vi "Arduino - Sensor shape data.vi"(8 "Error In":errorcluster, 10 "Sensor Data in":dbl[](array[numeric])) -> (0 "Error Out":errorcluster, 2 "Sensor Data Out":T1)   [LabVIEW 2014]
uses:
  Typedef/sensor_data.ctl
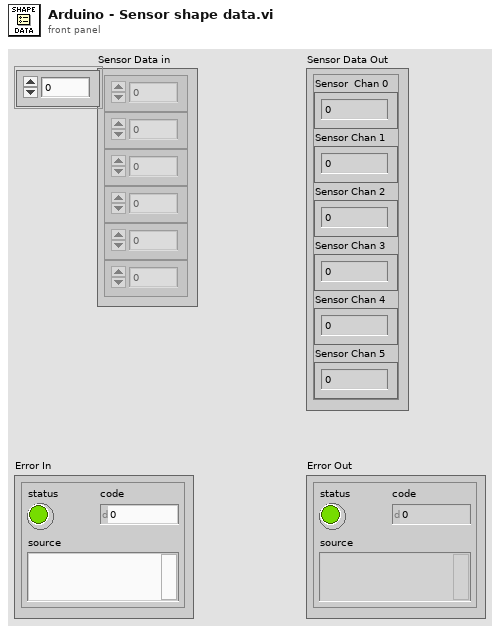
[diagram p1: front panel]
types:
  T1 = typedef "Sensor_data.ctl" = cluster{"Sensor  Chan 0":dbl, "Sensor Chan 1":dbl, "Sensor Chan 2":dbl, "Sensor Chan 3":dbl, "Sensor Chan 4":dbl, "Sensor Chan 5":dbl}
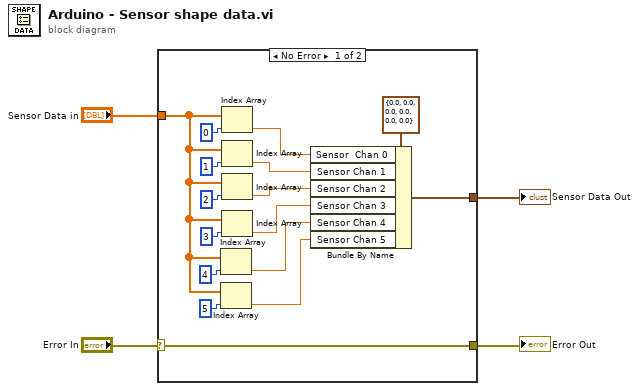
[diagram p0: block diagram]
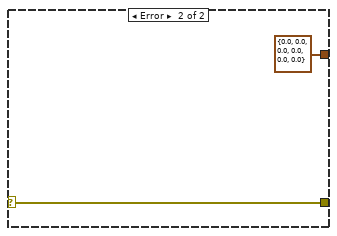
[diagram p2: hidden frame]
diagram:
  n1 = case shown="No Error" "Error In" {
    selector: "Error In" -> [w5 w21]
    tunnel: [w13 T1 {"Sensor  Chan 0"=0.0, "Sensor Chan 1"=0.0, "Sensor Chan 2"=0.0, "Sensor Chan 3"=0.0, "Sensor Chan 4"=0.0, "Sensor Chan 5"=0.0} ("Sensor Data")] -> w4
    tunnel: "Sensor Data in" -> [w12 _]
    tunnel: [w5 w21] -> w1
    frame No Error {
      n2 = Index Array(array=w12, index=4) -> (element=w7:dbl)
      n3 = Index Array(array=w12, index=5) -> (element=w6:dbl)
      n4 = Index Array(array=w12, index=0) -> (element=w11:dbl)
      n5 = Index Array(array=w12, index=1) -> (element=w10:dbl)
      n6 = Index Array(array=w12, index=2) -> (element=w9:dbl)
      n7 = Index Array(array=w12, index=3) -> (element=w8:dbl)
      n8 = Bundle By Name(cluster=T1 {"Sensor  Chan 0"=0.0, "Sensor Chan 1"=0.0, "Sensor Chan 2"=0.0, "Sensor Chan 3"=0.0, "Sensor Chan 4"=0.0, "Sensor Chan 5"=0.0} ("Sensor Data"), "Sensor  Chan 0"=w11, "Sensor Chan 1"=w10, "Sensor Chan 2"=w9, "Sensor Chan 3"=w8, "Sensor Chan 4"=w7, "Sensor Chan 5"=w6) -> (w13:T1)
    }
    frame Error {
    }
  }
  "Sensor Data Out" <- w4
  "Error Out" <- w1
